vi "Get Process Model.vi"(8 "error in (no error)":errorcluster, 11 "SequenceFile in":refnum<class "SequenceFile.lvclass">) -> (0 "error out":errorcluster, 2 "Process Model":refnum<class "SequenceFile.lvclass">, 3 "SequenceFile out":refnum<class "SequenceFile.lvclass">)   [LabVIEW 2020, in "TSnax.lvlib" / "SequenceFile.lvclass"]
uses:
  SequenceFile.lvclass
  C:/dev/illuminated-g/tsnax/TSnax/PropertyObjectFile/PropertyObjectFile.lvclass
  SequenceFile.lvclass/SequenceFile.ctl
  PropertyObject/PropertyObject.lvclass/PropertyObject.ctl
  PropertyObject/PropertyObject Ref.vi
  PropertyObjectFile/PropertyObjectFile.lvclass
  C:/dev/illuminated-g/tsnax/TSnax/PropertyObject/PropertyObject.lvclass
  PropertyObject/PropertyObject.lvclass
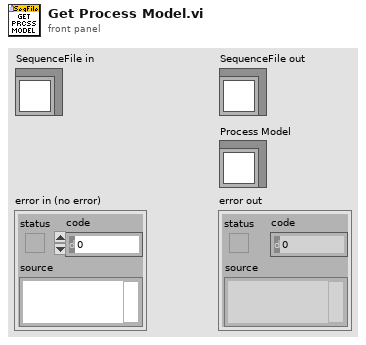
[diagram p1: front panel]
types:
  T1 = typedef "TSnax.lvlib/SequenceFile.lvclass/SequenceFile Type.ctl" = enum16{"Normal", "Model", "Front End Callbacks", "Station Callbacks", "Template"}
  T2 = typedef "TSnax.lvlib/SequenceFile.lvclass/Ref Data.ctl" = cluster{"Process Model":refnum<class "PropertyObjectFile.lvclass">, "File Globals":refnum<class "PropertyObject.lvclass">}
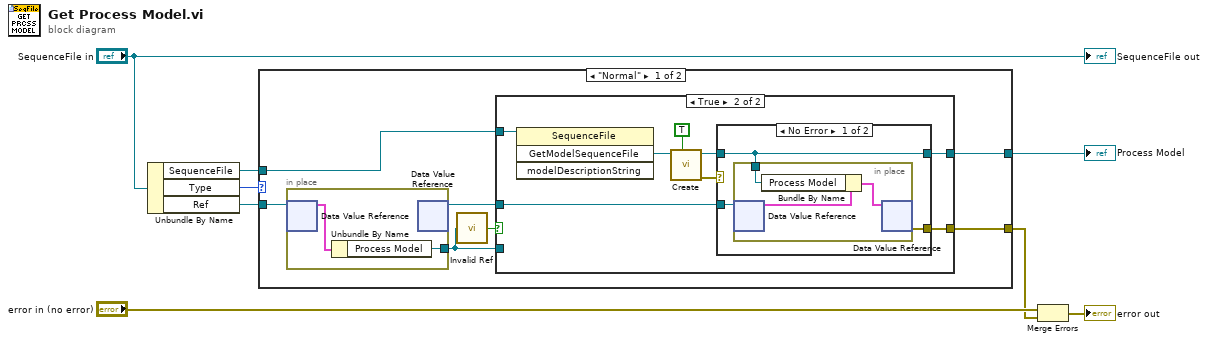
[diagram p0: block diagram]
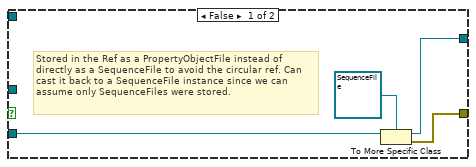
[diagram p2: hidden frame]
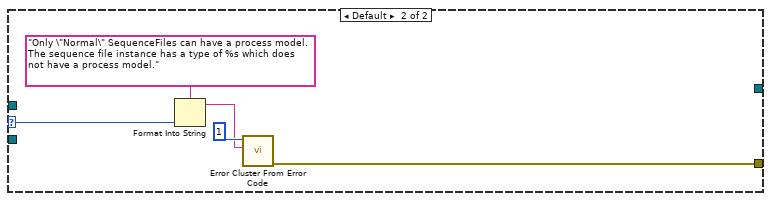
[diagram p4: hidden frame]
diagram:
  n1 = Unbundle By Name("SequenceFile in") -> ("SequenceFile"=w6:refnum<k7>, "Type"=w8:T1, "Ref"=w1:refnum<data-value>)
  n2 = case shown="\"Normal\"" w8 {
    selector: w8 -> [_ w40]
    tunnel: [w9 w37] -> w3
    tunnel: w1 -> [w15 _]
    tunnel: w6 -> [w12 _]
    tunnel: [w10 _] -> w5
    frame "Normal" {
      n3 = in-place {
        in-place-border: [w35] -> w13
        n4 = in-place-dvr #1(w15) -> (w36:T2)  [unwired: 1 out]
        n5 = Unbundle By Name(w36) -> ("Process Model"=w35:refnum<class "PropertyObjectFile.lvclass">)
        n6 = in-place-dvr #1() -> (w11:refnum<data-value>)  [unwired: 1 in, 1 out]
      }
      n7 = call "Invalid Ref.vi"("PropertyObject"=w13) -> ("Not a Valid Ref?"=w14:bool)
      n8 = case shown="True" w14 {
        tunnel: w13 -> [w19 _]
        tunnel: w12 -> [_ w27]
        tunnel: w11 -> [_ w25]
        tunnel: [w18 w21] -> w10
        tunnel: [w16 w22] -> w9
        frame False {
          # "Stored in the Ref as a PropertyObjectFile instead of directly as a SequenceFile to avoid the circular ref. Can cast it back to a SequenceFile instance since we can assume only SequenceFiles were stored."
          n9 = To More Specific Class(target class=refnum<class "SequenceFile.lvclass"> refnum ("TSnax.lvlib:SequenceFile.lvclass"), reference=w19) -> (specific class reference=w18:refnum<class "SequenceFile.lvclass">, error out=w16:errorcluster)  [unwired: 1 in]
        }
        frame True {
          n10 = invoke class="SequenceFile" method="GetModelSequenceFile"(reference=w27) -> ("GetModelSequenceFile"=w26:refnum<k7>)  [unwired: 3 in, 3 out]
          n11 = call "Create.vi"("Skip Unload? (F)"=TRUE, "SequenceFile"=w26) -> ("error out"=w24:errorcluster, "SequenceFile out"=w23:refnum<class "SequenceFile.lvclass">)  [unwired: 8 in]
          n12 = case shown="No Error" w24 {
            selector: w24 -> [_ w34]
            tunnel: w25 -> [w30 _]
            tunnel: w23 -> [w28 _]
            tunnel: [w29 w34] -> w22
            tunnel: [w28 _] -> w21
            frame No Error {
              n13 = in-place {
                in-place-border: w28 -> [w31]
                n14 = in-place-dvr #2(w30) -> (w33:T2)  [unwired: 1 out]
                n15 = Bundle By Name(cluster=w33, "Process Model"=w31) -> (w32:T2)
                n16 = in-place-dvr #2(w32) -> (w29:errorcluster)  [unwired: 1 out]
              }
            }
            frame Error {
            }
          }
        }
      }
    }
    frame Default {
      n17 = Format Into String(format string="Only \"Normal\" SequenceFiles can have a process model. The sequence file instance has a type of %s which does not have a process model.", w40) -> (resulting string=w38:string)  [unwired: 2 in, 1 out]
      n18 = call <vilib>:"Error Cluster From Error Code.vi"("error message (\"\")"=w38, "error code (0)"=1) -> ("error out"=w37:errorcluster)  [unwired: 7 in]
    }
  }
  "Process Model" <- w5
  n19 = Merge Errors("error in (no error)", w3) -> (→"error out":errorcluster)
  "SequenceFile out" <- "SequenceFile in"
